vi "Manual Save and Edit.vi"() -> ()   [LabVIEW 2015]
uses:
  <vilib>/Utility/config.llb/Write Key (String).vi
  <vilib>/Utility/config.llb/NI_LVConfig.lvlib
panel:
  in  "Preferences":string[][](array[string])
  in  "Cancel":bool
  in  "Save":bool
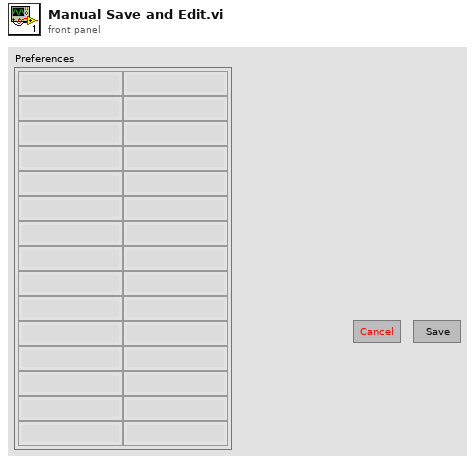
[diagram p1: front panel]
types:
  T1 = typedef "NI_LVConfig.lvlib/Config Data RefNum.ctl" = refnum<k1>
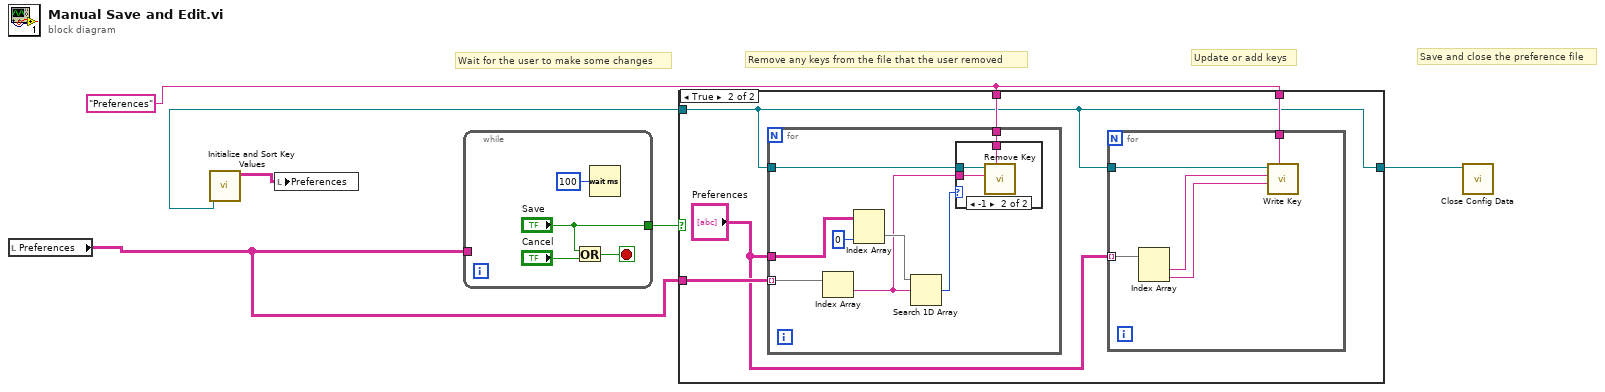
[diagram p0: block diagram]
diagram:
  w3 = "Preferences" ("section")
  # "Save and close the preference file"
  # "Update or add keys"
  # "Remove any keys from the file that the user removed"
  # "Wait for the user to make some changes"
  n1 = local read "Preferences"() -> (w2:string[][])
  n2 = call "Initialize and Sort Key Values.vi"() -> ("refnum"=w4:T1, "Preferences"=w1:string[][])  [unwired: 10 in]
  n3 = local write "Preferences"(w1) -> ()
  n4 = while {
    tunnel: ["Save"] -> w5
    tunnel: w2 -> [_]
    stop <- w9 stop-if-true
    n5 = Or(x="Save", y="Cancel") -> (x .or. y?=w9:bool)
    n6 = Wait (ms)(milliseconds to wait=u32 100) -> ()  [unwired: 1 out]
  }
  n7 = case shown="True" w5 {
    tunnel: w4 -> [w11 w13]
    tunnel: w2 -> [_ w16]
    tunnel: w3 -> [_ w15]
    tunnel: [w11 w13] -> w6
    tunnel: w3 -> [_ w14]
    frame False {
    }
    frame True {
      n8 = for {
        tunnel: w13 -> [w26]
        tunnel: w16 -> [w29] mode=indexing
        tunnel: w15 -> [w25]
        tunnel: "Preferences" -> [w22]
        n9 = Index Array(array=w29) -> (element=w24:string)  [unwired: 1 in]
        n10 = Index Array(array=w22, index (col)=0 ("disabled index (col)")) -> (element=w27:string[])  [unwired: 1 in]
        n11 = Search 1D Array(1D array=w27, element=w24) -> (index of element=w23:i32)  [unwired: 1 in]
        n12 = case shown="-1" w23 {
          tunnel: w26 -> [_ w32]
          tunnel: w25 -> [_ w31]
          tunnel: w24 -> [_ w30]
          frame 0, Default {
          }
          frame -1 {
            n13 = call <vilib>:"Remove Key.vi"("section"=w31, "key"=w30, "refnum"=w32) -> ()  [unwired: 6 in, 3 out]
          }
        }
      }
      n14 = for {
        tunnel: "Preferences" -> [w21] mode=indexing
        tunnel: w13 -> [w20]
        tunnel: w14 -> [w19]
        n15 = Index Array(array=w21) -> (element #1=w18:string, element #2=w17:string)  [unwired: 2 in]
        n16 = call-poly <vilib>:"Write Key.vi"("section"=w19, "value"=w17, "key"=w18, "refnum"=w20) -> ()  [unwired: 5 in, 3 out]
      }
    }
  }
  n17 = call <vilib>:"Close Config Data.vi"("refnum"=w6) -> ()  [unwired: 9 in, 2 out]
